vi "InitCAN.vi"(8 "error in (no error)":errorcluster, 10 "Channel Num":T1, 11 "CAN-NI in":refnum<class "CAN-NI.lvclass">) -> (0 "error out":errorcluster, 3 "CAN-NI out":refnum<class "CAN-NI.lvclass">)   [LabVIEW 2019, in "CAN-NI.lvlib" / "CAN-NI.lvclass"]
uses:
  CAN-NI.lvclass
  CAN-Interface/TypeDef/Def-ChannelNum.ctl
  <vilib>/xnet/xnet.llb/XNET Create Session (Frame Input Stream).vi
  <vilib>/xnet/xnet.llb/XNET Create Session (Frame Output Stream).vi
  CAN-Interface/Class-Interface.lvclass
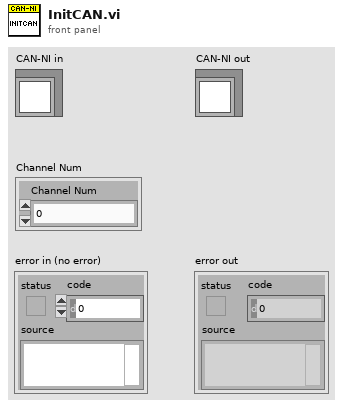
[diagram p1: front panel]
types:
  T1 = typedef "CAN-Interface.lvlib/Class-Interface.lvclass/Def-ChannelNum.ctl" = cluster{"Channel Num":u32}
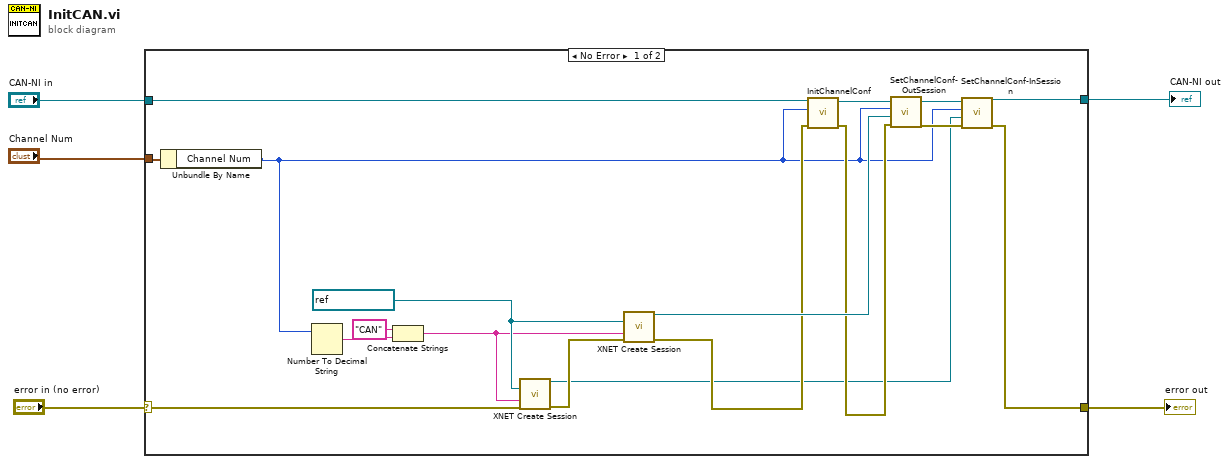
[diagram p0: block diagram]
diagram:
  n1 = case shown="No Error" "error in (no error)" {
    selector: "error in (no error)" -> [w15 w24]
    tunnel: "CAN-NI in" -> [w13 w25]
    tunnel: [w19 w25] -> w4
    tunnel: [w20 w24] -> w1
    tunnel: "Channel Num" -> [w7 _]
    frame No Error {
      w14 = refnum<k21> ":memory:" ("CAN Cluster")
      n2 = Unbundle By Name(w7) -> ("Channel Num"=w6:u32)
      n3 = Number To Decimal String(number=w6) -> (decimal integer string=w22:string)  [unwired: 1 in]
      n4 = Concatenate Strings("CAN" ("string"), w22) -> (w9:string)
      n5 = call-poly <vilib>:"XNET Create Session.vi"("cluster (:memory:)"=w14, "interface"=w9, "error in (no error)"=w15) -> ("session out"=w8:refnum<k21>, "error out"=w17:errorcluster)  [unwired: 11 in]
      n6 = call-poly <vilib>:"XNET Create Session.vi"("cluster (:memory:)"=w14, "interface"=w9, "error in (no error)"=w17) -> ("session out"=w18:refnum<k21>, "error out"=w12:errorcluster)  [unwired: 11 in]
      n7 = call "InitChannelConf.vi"("error in"=w12, "Channel Num"=w6, "CAN-NI"=w13) -> ("error out"=w11:errorcluster, "CAN-NI"=w10:refnum<class "CAN-NI.lvclass">)  [unwired: 7 in]
      n8 = call "SetChannelConf-OutSession.vi"("error in"=w11, "Out Session"=w18, "Channel Num"=w6, "CAN-NI"=w10) -> ("error out"=w16:errorcluster, "CAN-NI"=w21:refnum<class "CAN-NI.lvclass">)  [unwired: 6 in]
      n9 = call "SetChannelConf-InSession.vi"("error in"=w16, "In Session"=w8, "Channel Num"=w6, "CAN-NI"=w21) -> ("error out"=w20:errorcluster, "CAN-NI"=w19:refnum<class "CAN-NI.lvclass">)  [unwired: 6 in]
    }
    frame Error {
    }
  }
  "error out" <- w1
  "CAN-NI out" <- w4
